vi "RANGE Header Banks.vi"(5 "Meter":string, 11 "All Meter Data":T1) -> (3 "Header":string[](array[string]))   [LabVIEW 2018]
uses:
  Type Definitions/RANGE DAQ Data Four Meters.ctl
  Type Definitions/RANGE DAQ Data.ctl
  Drivers/Omega FMA-1600A Series Gas Flow Meter/Type Definitions/FMA1600A Gas Type.ctl
  Drivers/Omega FMA-1600A Series Gas Flow Meter/Type Definitions/FMA1600A Units String.ctl
  Type Definitions/RANGE GAS Data.ctl
  Type Definitions/RANGE Panel Data.ctl
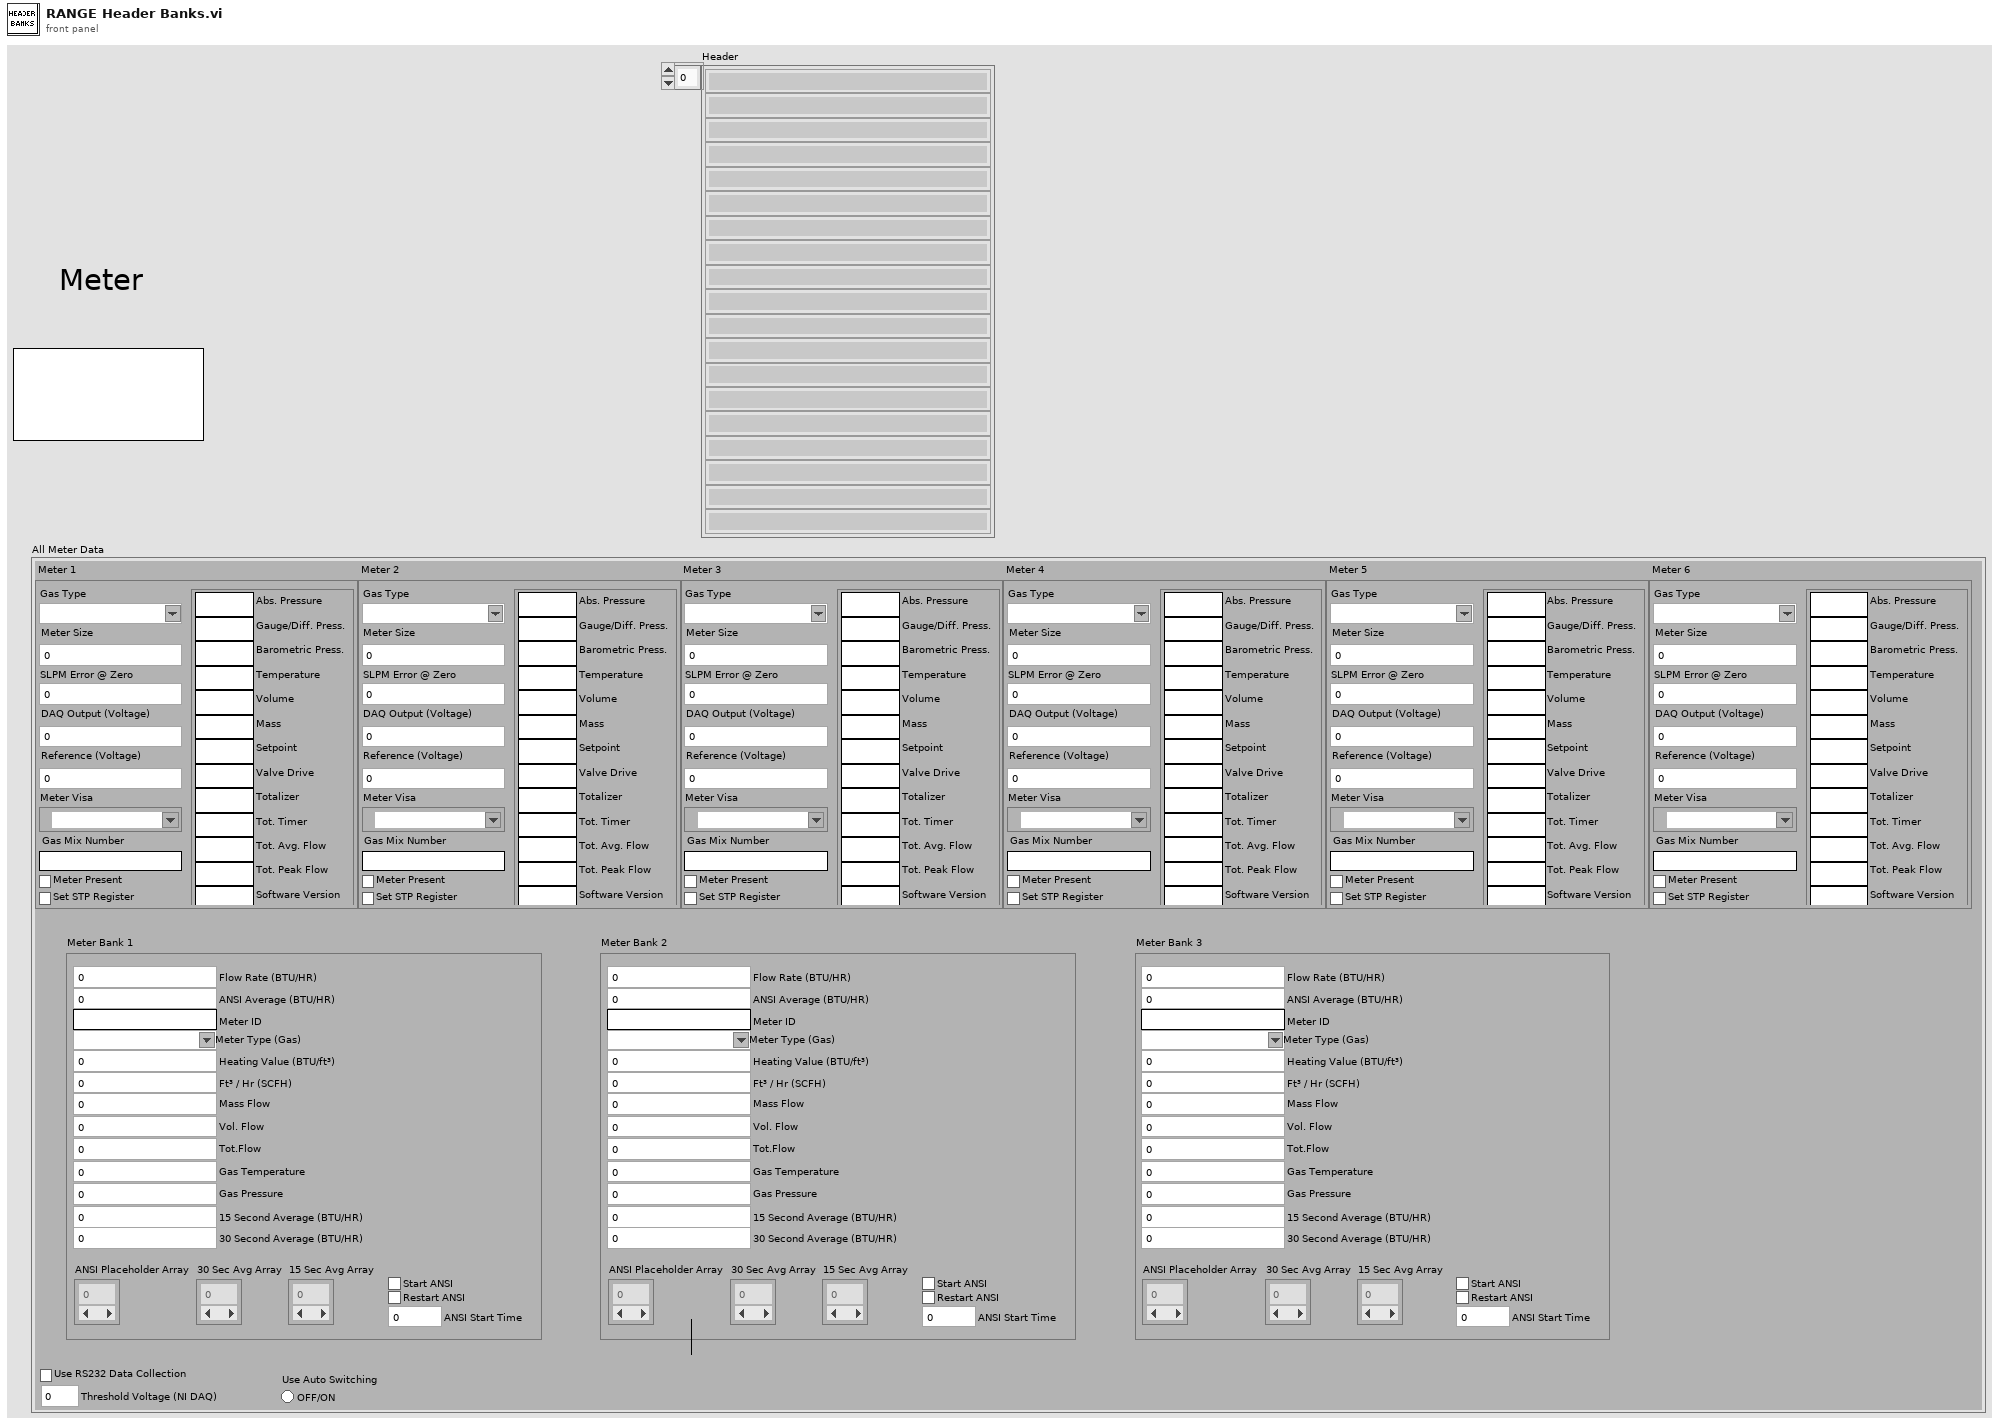
[diagram p1: front panel]
types:
  T1 = typedef "RANGE DAQ Data Four Meters.ctl" = cluster{"Meter 1":T2, "Meter 2":T2, "Meter 3":T2, "Meter 4":T2, "Meter 5":T2, "Meter 6":T2, "Meter Bank 1":T5, "Meter Bank 2":T5, "Meter Bank 3":T5, "Threshold Voltage (NI DAQ)":dbl, "Use RS232 Data Collection":bool, "Use Auto Switching":bool}
  T2 = typedef "RANGE DAQ Data.ctl" = cluster{"Meter Size":dbl, "DAQ Output (Voltage)":dbl, "Reference (Voltage)":dbl, "Meter Present":bool, "Meter Visa":refnum<visa-resource-name>, "Gas Type":T3, "SLPM Error @ Zero":dbl, "Gas Mix Number":string, "Set STP Register":bool, "Measurement Units":T4}
  T3 = typedef "FMA1600A Gas Type.ctl" = string
  T4 = typedef "FMA1600A Units String.ctl" = cluster{"Abs. Pressure":string, "Gauge/Diff. Press.":string, "Barometric Press.":string, "Temperature":string, "Volume":string, "Mass":string, "Setpoint":string, "Valve Drive":string, "Totalizer":string, "Tot. Timer":string, "Tot. Avg. Flow":string, "Tot. Peak Flow":string, "Software Version":string}
  T5 = typedef "RANGE GAS Data.ctl" = cluster{"Flow Rate (BTU/HR)":dbl, "ANSI Placeholder Array":dbl[], "15 Sec Avg Array":dbl[], "30 Sec Avg Array ":dbl[], "ANSI Average (BTU/HR)":dbl, "Panel Data":T6, "Start ANSI":bool, "ANSI Start Time":dbl, "Restart ANSI":bool, "Meter ID":string}
  T6 = typedef "RANGE Panel Data.ctl" = cluster{"Meter Type (Gas)":T3, "Heating Value (BTU/ft³)":dbl, "Ft³ / Hr (SCFH)":dbl, "15 Second Average (BTU/HR)":dbl, "30 Second Average (BTU/HR)":dbl, "Mass Flow":dbl, "Vol. Flow":dbl, "Gas Temperature":dbl, "Gas Pressure":dbl, "Tot.Flow":dbl}
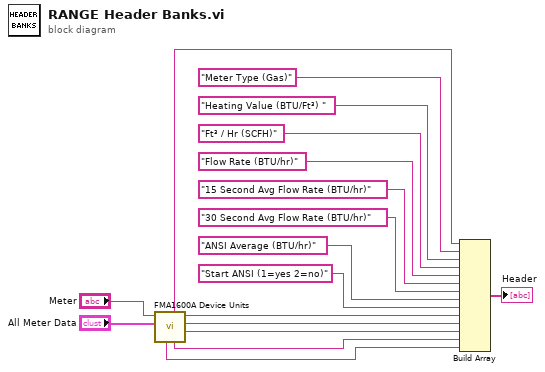
[diagram p0: block diagram]
diagram:
  n1 = call "FMA1600A Device Units.vi"("All Meter Data"="All Meter Data", "Meter"="Meter") -> ("Gas Temperature"=w14:string, "Vol. Flow-Measured"=w13:string, "Mass Flow-Measured"=w11:string, "Gas Pressure"=w15:string, "Gas Meter ID"=w1:string, "Totalized Flow"=w16:string)  [unwired: 3 in, 1 out]
  n2 = Build Array(w1, "Meter Type (Gas)", "Heating Value (BTU/Ft³) ", "Ft³ / Hr (SCFH)", "Flow Rate (BTU/hr)", "15 Second Avg Flow Rate (BTU/hr)", "30 Second Avg Flow Rate (BTU/hr)", "ANSI Average (BTU/hr)", "Start ANSI (1=yes 2=no)", w11, w13, w14, w15, w16) -> (→"Header":string[])
